vi "pumonarytesting_auto.vi"() -> ()   [LabVIEW 2014]
uses:
  <vilib>/vision/NI_Vision_Development_Module.lvlib
  <instrlib>/KD Scientific 2XX Series/KD Scientific 2XX Series.lvlib
panel:
  in  "Number of Cycles":i32
  out "Status":T1
  in  "stop 2":bool
  out "Delivered Volume":dbl
  out "Units":string
  in  "number of steps":i32
  in  "Baud Rate (9600)":u32(ring)=9600 items=["300"=300, "1200"=1200, "2400"=2400, "4800"=4800, "9600"=9600]
  in  "Withdrawal Settings":T2={"Flow Rate (5)"=5.0, "Volume (10)"=10.0, "Volume Units (ml)"=enum."milliliters (ml)", "Rate Units (ml/min.)"=enum."milliliters per minute (ml/min.)"} {"Volume (10)" format="%#.3g"}
  in  "Diameter (8.75 mm)":dbl=8.75
  in  "Infusion Settings":T2={"Flow Rate (5)"=5.0, "Volume (10)"=10.0, "Volume Units (ml)"=enum."milliliters (ml)", "Rate Units (ml/min.)"=enum."milliliters per minute (ml/min.)"}
  in  "Address (0)":i32 format="%0.0f"
  in  "error in (no error)":errorcluster
  in  "VISA resource name":refnum<visa-resource-name>="COM1"
  in  "stop 4":bool
  in  "stop":bool
  out "Image":T3(plugin-control)
  out "Particle Measurements (Pixels) (Particle Analysis 1)":dbl[][](array[numeric]) format="%.2f"
  out "subarray":dbl[](array[numeric])
  out "The diameter":dbl[](array[numeric])
  in  "stop (F)":bool
  out "Data from Transducer":dynamicdata(graph) caption="Voltage from Transducer V"
  out "Voltage from pressure transducer":dbl[](array[numeric])
  out "Pressure mm Hg":dbl[](graph)
  in  "Calibration factor":dbl[](array[numeric])
  in  "Zero Error":dbl[](array[numeric])
  out "pressure mm Hg":dbl[](array[numeric])
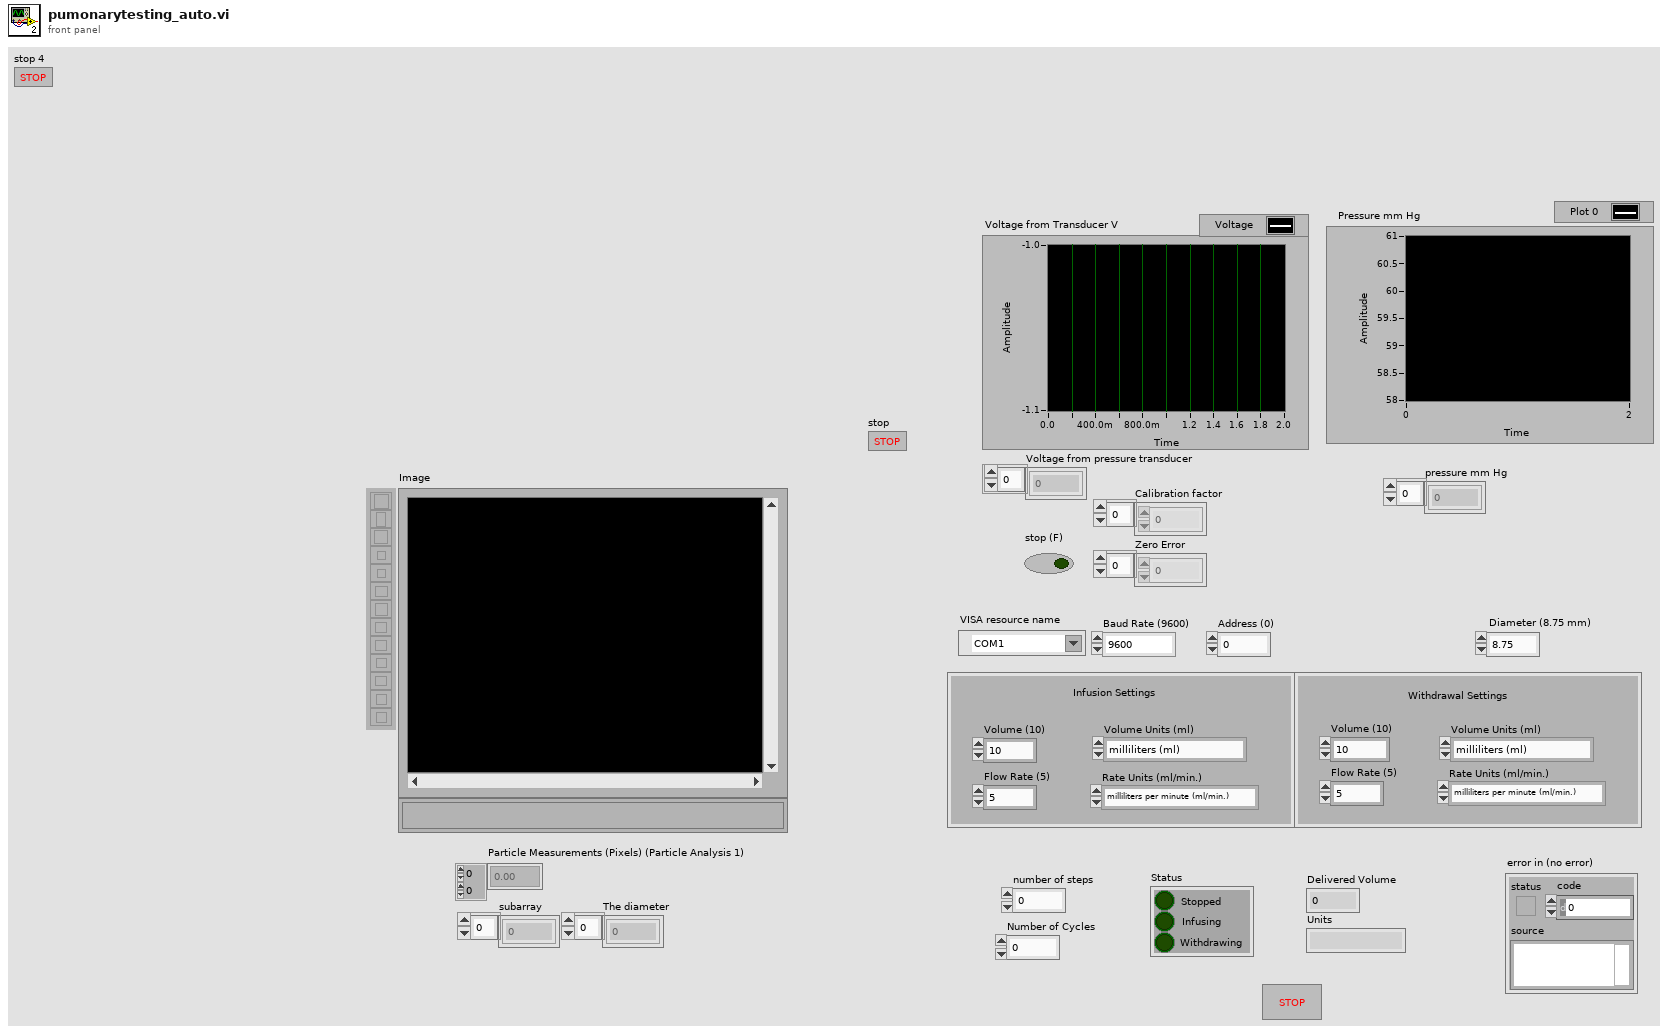
[diagram p1: front panel]
types:
  T1 = cluster{"Stopped":bool, "Infusing":bool, "Withdrawing":bool}
  T2 = cluster{"Flow Rate (5)":dbl, "Volume (10)":dbl, "Volume Units (ml)":enum16{"milliliters (ml)", "microliters (ul)"}, "Rate Units (ml/min.)":enum16{"milliliters per minute (ml/min.)", "milliliters per hour (ml/hr.)", "microliters per minute (ul/min.)", "microliters per hour (ul/hr.)"}}
  T3 = typedef "IMAQ Image.ctl" = refnum<image>
  T4 = typedef "Board Id" = u8
  T5 = typedef "ROI Descriptor" = cluster{"Global Rectangle":i32[], "Contours":cluster{"ID":enum32{"External", "Internal"}, "Type":u32, "Coordinates":i32[]}[]}
  T6 = enum16{"milliliters per minute (ml/min.)", "milliliters per hour (ml/hr.)", "microliters per minute (ul/min.)", "microliters per hour (ul/hr.)"}
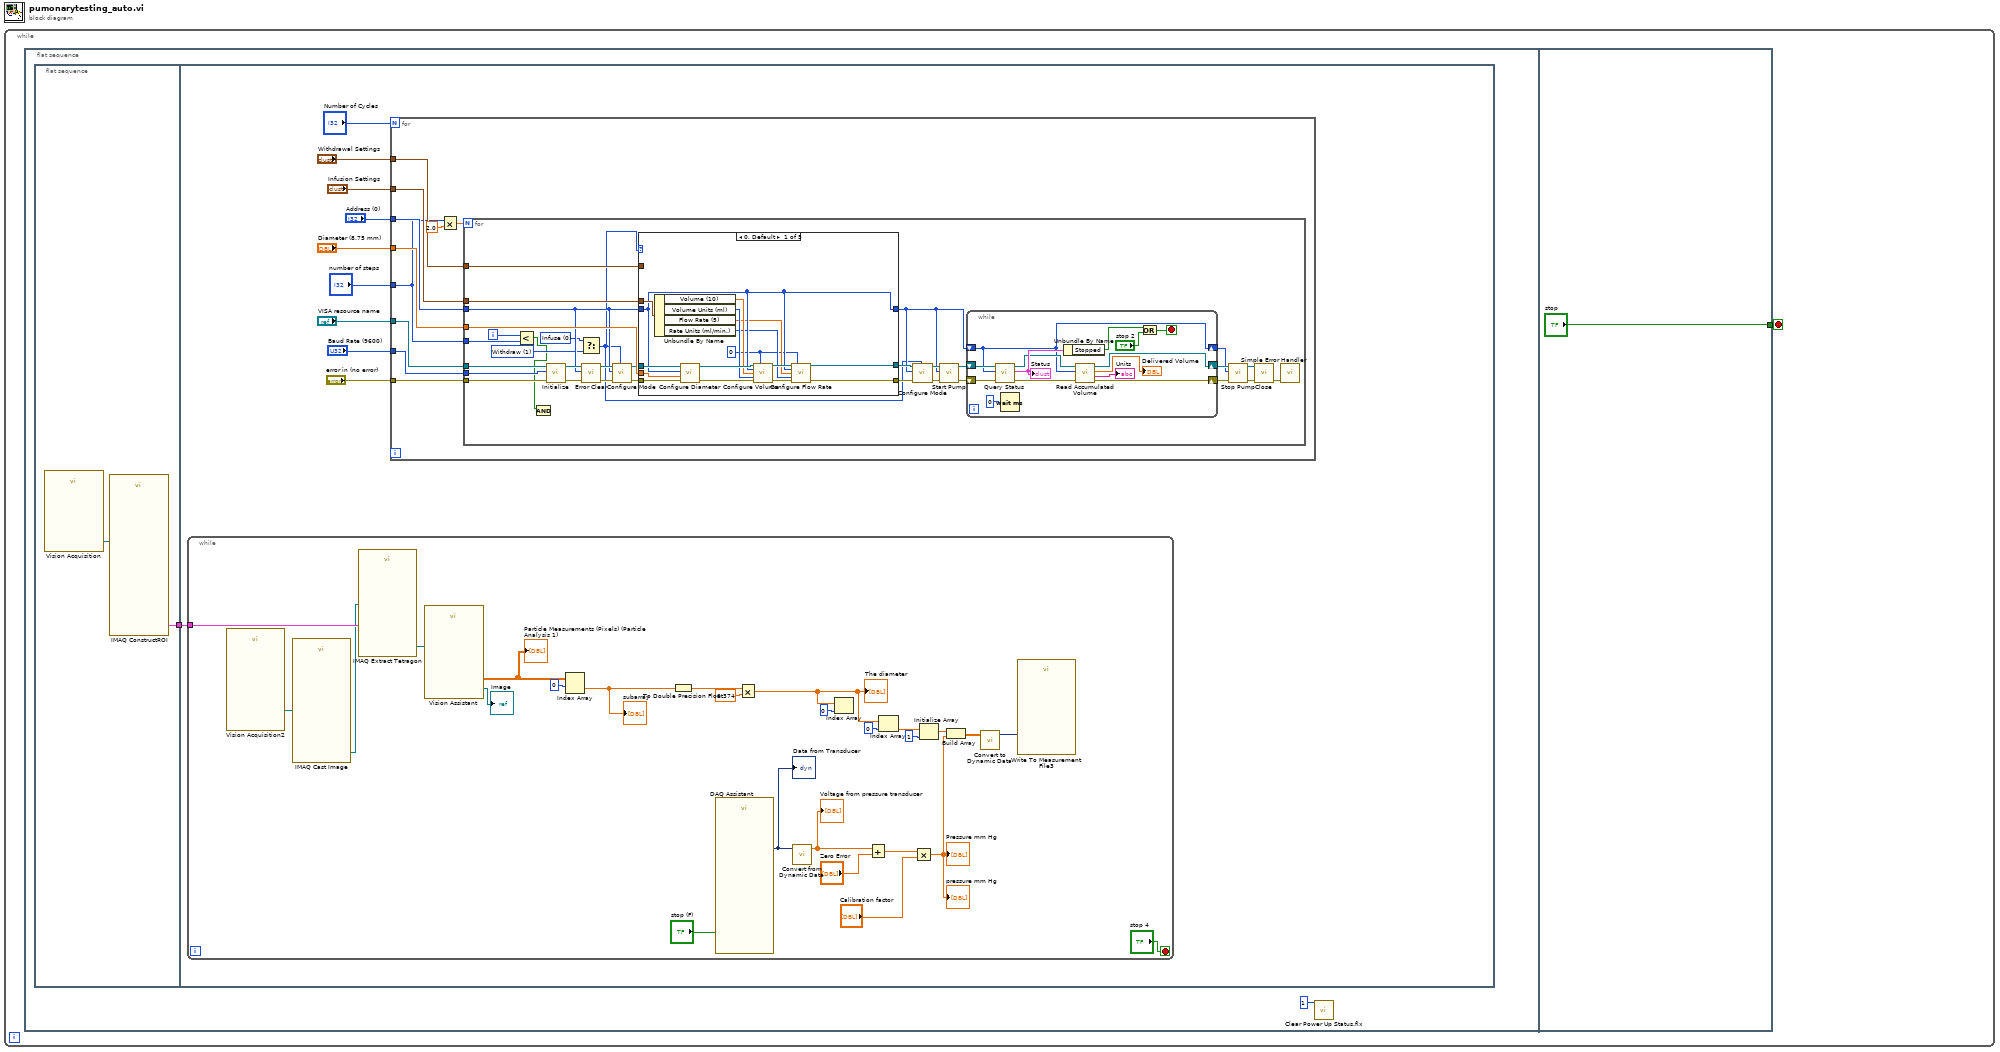
[diagram p0: block diagram]
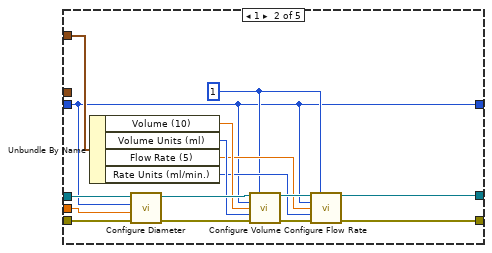
[diagram p2: hidden frame]
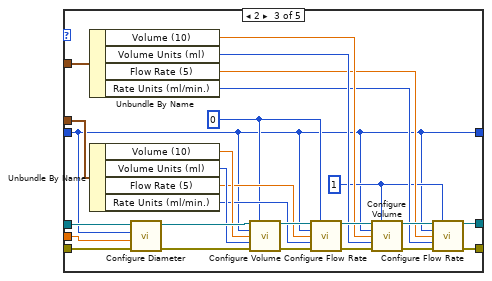
[diagram p3: hidden frame]
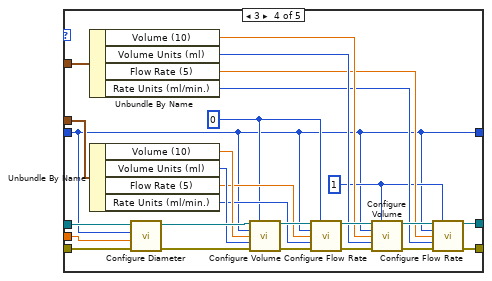
[diagram p4: hidden frame]
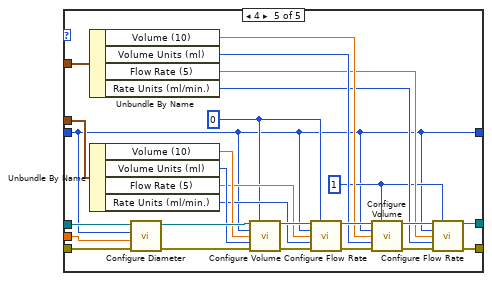
[diagram p5: hidden frame]
diagram:
  n1 = while {
    stop <- w1 stop-if-true
    n2 = flat-sequence {
      tunnel: ["stop"] -> w1
      frame #0 {
        n3 = flat-sequence {
          tunnel: [w4] -> w3
          tunnel: w3 -> [w15]
          frame #0 {
            n4 = call "Vision Acquisition"() -> ("Image Out"=w5:T3)  [unwired: 26 in, 1 out]
            n5 = call "IMAQ ConstructROI"("Image"=w5) -> ("ROI Descriptor Out"=w4:T5)  [unwired: 7 in, 3 out]
          }
          frame #1 {
            n6 = while {
              tunnel: w15 -> [w207]
              stop <- "stop 4" stop-if-true
              n7 = call "Vision Acquisition2"() -> ("Image Out"=w191:T3)  [unwired: 25 in, 2 out]
              n8 = call "IMAQ Cast Image"("Image Src"=w191) -> ("Image Dst Out"=w198:T3)  [unwired: 9 in, 1 out]
              n9 = call-poly "IMAQ Extract Tetragon"("ROI Descriptor"=w207, "Image Src"=w198) -> ("Image Dst Out"=w199:T3)  [unwired: 8 in, 1 out]
              n10 = call "Vision Assistant"("Image In"=w199) -> ("Image Out"=→"Image":T3, "Particle Measurements (Pixels) (Particle Analysis 1)"=w197:dbl[][])  [unwired: 23 in, 2 out]
              "Particle Measurements (Pixels) (Particle Analysis 1)" <- w197
              n11 = Index Array(array=w197, index (row)=0) -> (element=w195:dbl[])  [unwired: 1 in]
              "subarray" <- w195
              n12 = To Double Precision Float(number=w195) -> (double precision float=w194:dbl[])
              n13 = call "DAQ Assistant"("stop (F)"="stop (F)") -> ("data"=w206:dynamicdata)  [unwired: 15 in, 3 out]
              "Data from Transducer" <- w206
              n14 = Multiply(x=w194, y=0.374) -> (x*y=w187:dbl[])
              "The diameter" <- w187
              n15 = call "Convert from Dynamic Data"("Dynamic Data Type"=w206) -> ("Array"=w203:dbl[])  [unwired: 3 in]
              "Voltage from pressure transducer" <- w203
              n16 = Index Array(array=w187, index=0) -> ()  [unwired: 1 out]
              n17 = Add(x=w203, y="Zero Error") -> (x+y=w205:dbl[])
              n18 = Index Array(array=w187, index=0) -> (element=w186:dbl)
              n19 = Multiply(x=w205, y="Calibration factor") -> (x*y=w189:dbl[])
              "Pressure mm Hg" <- w189
              "pressure mm Hg" <- w189
              n20 = Initialize Array(w186, 1 ("dimension size")) -> (w184:dbl[])
              n21 = Build Array(w184, w189) -> (w183:dbl[][])
              n22 = call "Convert to Dynamic Data"("2D Array"=w183) -> ("Dynamic Data Type"=w182:dynamicdata)  [unwired: 3 in]
              n23 = call "Write To Measurement File3"("Signals"=w182) -> ()  [unwired: 16 in, 3 out]
            }
            n24 = for {
              N: "Number of Cycles" -> [_]
              tunnel: "VISA resource name" -> [w25]
              tunnel: "error in (no error)" -> [w24]
              tunnel: "Infusion Settings" -> [w23]
              tunnel: "Withdrawal Settings" -> [w22]
              tunnel: "Diameter (8.75 mm)" -> [w21]
              tunnel: "Baud Rate (9600)" -> [w20]
              tunnel: "Address (0)" -> [w19]
              tunnel: "number of steps" -> [w16]
              n25 = Multiply(x=w16, y=2.0) -> (x*y=w17:dbl)
              n26 = for {
                N: w17 -> [_]
                tunnel: w25 -> [w57]
                tunnel: w24 -> [w56]
                tunnel: w23 -> [w51]
                tunnel: w22 -> [w50]
                tunnel: w21 -> [w49]
                tunnel: w20 -> [w44]
                tunnel: w19 -> [w32]
                tunnel: w16 -> [w30]
                i -> [w31]
                w28 = u16 1 items=["Withdraw"=1]
                w29 = u16 0 items=["Infuse"] ("Mode (infuse)")
                n27 = Less?(x=w31, y=w30) -> (x < y?=w26:bool)
                n28 = And(x=w26) -> ()  [unwired: 1 in, 1 out]
                n29 = call <instrlib>:"Initialize.vi"("error in (no error)"=w56, "Baud Rate (9600)"=w44, "VISA resource name"=w57) -> ("error out"=w34:errorcluster, "VISA resource name out"=w33:refnum<visa-resource-name>)  [unwired: 7 in]
                n30 = Select(t=w29, f=w28) -> (s? t:f=w27:u16)  [unwired: 1 in]
                n31 = call <instrlib>:"Error Clear.vi"("error in (no error)"=w34, "Address (0)"=w32, "VISA resource name"=w33) -> ("error out"=w35:errorcluster, "VISA resource name out"=w36:refnum<visa-resource-name>)  [unwired: 6 in, 1 out]
                n32 = call <instrlib>:"Configure Mode.vi"("Mode (infuse)"=w27, "error in (no error)"=w35, "Address (0)"=w32, "VISA resource name"=w36) -> ("error out"=w38:errorcluster, "VISA resource name out"=w37:refnum<visa-resource-name>)  [unwired: 6 in]
                n33 = case shown="0, Default" w27 {
                  tunnel: w51 -> [w67 _ w115 w141 w167]
                  tunnel: w50 -> [_ w89 w114 w140 w166]
                  tunnel: w37 -> [w73 w88 w113 w139 w165]
                  tunnel: w38 -> [w72 w84 w112 w138 w164]
                  tunnel: w49 -> [w66 w80 w95 w121 w147]
                  tunnel: [w65 w74 w90 w116 w142] -> w39
                  tunnel: w32 -> [w65 w74 w90 w116 w142]
                  tunnel: [w60 w85 w92 w118 w144] -> w43
                  tunnel: [w59 w81 w91 w117 w143] -> w42
                  frame 0, Default {
                    w58 = 0
                    n34 = Unbundle By Name(w67) -> ("Volume (10)"=w64:dbl, "Volume Units (ml)"=w63:enum16{"milliliters (ml)", "microliters (ul)"}, "Flow Rate (5)"=w62:dbl, "Rate Units (ml/min.)"=w61:T6)
                    n35 = call <instrlib>:"Configure Diameter.vi"("error in (no error)"=w72, "Diameter (8.75 mm)"=w66, "Address (0)"=w65, "VISA resource name"=w73) -> ("error out"=w70:errorcluster, "VISA resource name out"=w71:refnum<visa-resource-name>)  [unwired: 6 in]
                    n36 = call <instrlib>:"Configure Volume.vi"("VISA resource name"=w71, "Mode (infuse)"=w58, "Address (0)"=w65, "Volume (100)"=w64, "Units (0: milliliters)"=w63, "error in (no error)"=w70) -> ("VISA resource name out"=w69:refnum<visa-resource-name>, "error out"=w68:errorcluster)  [unwired: 8 in]
                    n37 = call <instrlib>:"Configure Flow Rate.vi"("VISA resource name"=w69, "Mode (infuse)"=w58, "Address (0)"=w65, "Flow Rate (5)"=w62, "Units (0: milliliters per minute)"=w61, "error in (no error)"=w68) -> ("VISA resource name out"=w60:refnum<visa-resource-name>, "error out"=w59:errorcluster)  [unwired: 8 in]
                  }
                  frame 1 {
                    w75 = 1
                    n38 = Unbundle By Name(w89) -> ("Volume (10)"=w79:dbl, "Volume Units (ml)"=w78:enum16{"milliliters (ml)", "microliters (ul)"}, "Flow Rate (5)"=w77:dbl, "Rate Units (ml/min.)"=w76:T6)
                    n39 = call <instrlib>:"Configure Diameter.vi"("error in (no error)"=w84, "Diameter (8.75 mm)"=w80, "Address (0)"=w74, "VISA resource name"=w88) -> ("error out"=w83:errorcluster, "VISA resource name out"=w87:refnum<visa-resource-name>)  [unwired: 6 in]
                    n40 = call <instrlib>:"Configure Volume.vi"("VISA resource name"=w87, "Mode (infuse)"=w75, "Address (0)"=w74, "Volume (100)"=w79, "Units (0: milliliters)"=w78, "error in (no error)"=w83) -> ("VISA resource name out"=w86:refnum<visa-resource-name>, "error out"=w82:errorcluster)  [unwired: 8 in]
                    n41 = call <instrlib>:"Configure Flow Rate.vi"("VISA resource name"=w86, "Mode (infuse)"=w75, "Address (0)"=w74, "Flow Rate (5)"=w77, "Units (0: milliliters per minute)"=w76, "error in (no error)"=w82) -> ("VISA resource name out"=w85:refnum<visa-resource-name>, "error out"=w81:errorcluster)  [unwired: 8 in]
                  }
                  frame 2 {
                    w93 = 1
                    w94 = 0
                    n42 = Unbundle By Name(w114) -> ("Volume (10)"=w99:dbl, "Volume Units (ml)"=w98:enum16{"milliliters (ml)", "microliters (ul)"}, "Flow Rate (5)"=w97:dbl, "Rate Units (ml/min.)"=w96:T6)
                    n43 = Unbundle By Name(w115) -> ("Volume (10)"=w103:dbl, "Volume Units (ml)"=w102:enum16{"milliliters (ml)", "microliters (ul)"}, "Flow Rate (5)"=w101:dbl, "Rate Units (ml/min.)"=w100:T6)
                    n44 = call <instrlib>:"Configure Diameter.vi"("error in (no error)"=w112, "Diameter (8.75 mm)"=w95, "Address (0)"=w90, "VISA resource name"=w113) -> ("error out"=w107:errorcluster, "VISA resource name out"=w111:refnum<visa-resource-name>)  [unwired: 6 in]
                    n45 = call <instrlib>:"Configure Volume.vi"("VISA resource name"=w111, "Mode (infuse)"=w94, "Address (0)"=w90, "Volume (100)"=w103, "Units (0: milliliters)"=w102, "error in (no error)"=w107) -> ("VISA resource name out"=w110:refnum<visa-resource-name>, "error out"=w106:errorcluster)  [unwired: 8 in]
                    n46 = call <instrlib>:"Configure Flow Rate.vi"("VISA resource name"=w110, "Mode (infuse)"=w94, "Address (0)"=w90, "Flow Rate (5)"=w101, "Units (0: milliliters per minute)"=w100, "error in (no error)"=w106) -> ("VISA resource name out"=w109:refnum<visa-resource-name>, "error out"=w105:errorcluster)  [unwired: 8 in]
                    n47 = call <instrlib>:"Configure Volume.vi"("VISA resource name"=w109, "Mode (infuse)"=w93, "Address (0)"=w90, "Volume (100)"=w99, "Units (0: milliliters)"=w98, "error in (no error)"=w105) -> ("VISA resource name out"=w108:refnum<visa-resource-name>, "error out"=w104:errorcluster)  [unwired: 8 in]
                    n48 = call <instrlib>:"Configure Flow Rate.vi"("VISA resource name"=w108, "Mode (infuse)"=w93, "Address (0)"=w90, "Flow Rate (5)"=w97, "Units (0: milliliters per minute)"=w96, "error in (no error)"=w104) -> ("VISA resource name out"=w92:refnum<visa-resource-name>, "error out"=w91:errorcluster)  [unwired: 8 in]
                  }
                  frame 3 {
                    w119 = 1
                    w120 = 0
                    n49 = Unbundle By Name(w140) -> ("Volume (10)"=w125:dbl, "Volume Units (ml)"=w124:enum16{"milliliters (ml)", "microliters (ul)"}, "Flow Rate (5)"=w123:dbl, "Rate Units (ml/min.)"=w122:T6)
                    n50 = Unbundle By Name(w141) -> ("Volume (10)"=w129:dbl, "Volume Units (ml)"=w128:enum16{"milliliters (ml)", "microliters (ul)"}, "Flow Rate (5)"=w127:dbl, "Rate Units (ml/min.)"=w126:T6)
                    n51 = call <instrlib>:"Configure Diameter.vi"("error in (no error)"=w138, "Diameter (8.75 mm)"=w121, "Address (0)"=w116, "VISA resource name"=w139) -> ("error out"=w133:errorcluster, "VISA resource name out"=w137:refnum<visa-resource-name>)  [unwired: 6 in]
                    n52 = call <instrlib>:"Configure Volume.vi"("VISA resource name"=w137, "Mode (infuse)"=w120, "Address (0)"=w116, "Volume (100)"=w129, "Units (0: milliliters)"=w128, "error in (no error)"=w133) -> ("VISA resource name out"=w136:refnum<visa-resource-name>, "error out"=w132:errorcluster)  [unwired: 8 in]
                    n53 = call <instrlib>:"Configure Flow Rate.vi"("VISA resource name"=w136, "Mode (infuse)"=w120, "Address (0)"=w116, "Flow Rate (5)"=w127, "Units (0: milliliters per minute)"=w126, "error in (no error)"=w132) -> ("VISA resource name out"=w135:refnum<visa-resource-name>, "error out"=w131:errorcluster)  [unwired: 8 in]
                    n54 = call <instrlib>:"Configure Volume.vi"("VISA resource name"=w135, "Mode (infuse)"=w119, "Address (0)"=w116, "Volume (100)"=w125, "Units (0: milliliters)"=w124, "error in (no error)"=w131) -> ("VISA resource name out"=w134:refnum<visa-resource-name>, "error out"=w130:errorcluster)  [unwired: 8 in]
                    n55 = call <instrlib>:"Configure Flow Rate.vi"("VISA resource name"=w134, "Mode (infuse)"=w119, "Address (0)"=w116, "Flow Rate (5)"=w123, "Units (0: milliliters per minute)"=w122, "error in (no error)"=w130) -> ("VISA resource name out"=w118:refnum<visa-resource-name>, "error out"=w117:errorcluster)  [unwired: 8 in]
                  }
                  frame 4 {
                    w145 = 1
                    w146 = 0
                    n56 = Unbundle By Name(w166) -> ("Volume (10)"=w151:dbl, "Volume Units (ml)"=w150:enum16{"milliliters (ml)", "microliters (ul)"}, "Flow Rate (5)"=w149:dbl, "Rate Units (ml/min.)"=w148:T6)
                    n57 = Unbundle By Name(w167) -> ("Volume (10)"=w155:dbl, "Volume Units (ml)"=w154:enum16{"milliliters (ml)", "microliters (ul)"}, "Flow Rate (5)"=w153:dbl, "Rate Units (ml/min.)"=w152:T6)
                    n58 = call <instrlib>:"Configure Diameter.vi"("error in (no error)"=w164, "Diameter (8.75 mm)"=w147, "Address (0)"=w142, "VISA resource name"=w165) -> ("error out"=w159:errorcluster, "VISA resource name out"=w163:refnum<visa-resource-name>)  [unwired: 6 in]
                    n59 = call <instrlib>:"Configure Volume.vi"("VISA resource name"=w163, "Mode (infuse)"=w146, "Address (0)"=w142, "Volume (100)"=w155, "Units (0: milliliters)"=w154, "error in (no error)"=w159) -> ("VISA resource name out"=w162:refnum<visa-resource-name>, "error out"=w158:errorcluster)  [unwired: 8 in]
                    n60 = call <instrlib>:"Configure Flow Rate.vi"("VISA resource name"=w162, "Mode (infuse)"=w146, "Address (0)"=w142, "Flow Rate (5)"=w153, "Units (0: milliliters per minute)"=w152, "error in (no error)"=w158) -> ("VISA resource name out"=w161:refnum<visa-resource-name>, "error out"=w157:errorcluster)  [unwired: 8 in]
                    n61 = call <instrlib>:"Configure Volume.vi"("VISA resource name"=w161, "Mode (infuse)"=w145, "Address (0)"=w142, "Volume (100)"=w151, "Units (0: milliliters)"=w150, "error in (no error)"=w157) -> ("VISA resource name out"=w160:refnum<visa-resource-name>, "error out"=w156:errorcluster)  [unwired: 8 in]
                    n62 = call <instrlib>:"Configure Flow Rate.vi"("VISA resource name"=w160, "Mode (infuse)"=w145, "Address (0)"=w142, "Flow Rate (5)"=w149, "Units (0: milliliters per minute)"=w148, "error in (no error)"=w156) -> ("VISA resource name out"=w144:refnum<visa-resource-name>, "error out"=w143:errorcluster)  [unwired: 8 in]
                  }
                }
                n63 = call <instrlib>:"Configure Mode.vi"("Mode (infuse)"=w27, "error in (no error)"=w42, "Address (0)"=w39, "VISA resource name"=w43) -> ("error out"=w40:errorcluster, "VISA resource name out"=w41:refnum<visa-resource-name>)  [unwired: 6 in]
                n64 = call <instrlib>:"Start Pump.vi"("error in (no error)"=w40, "Address (0)"=w39, "VISA resource name"=w41) -> ("error out"=w54:errorcluster, "VISA resource name out"=w55:refnum<visa-resource-name>)  [unwired: 7 in]
                n65 = while {
                  shift-right: [w170] -> w48
                  shift-left: w39 -> [w170]
                  shift-right: [w172] -> w53
                  shift-left: w55 -> [w178]
                  shift-right: [w171] -> w52
                  shift-left: w54 -> [w179]
                  stop <- w176 stop-if-true
                  n66 = call <instrlib>:"Query Status.vi"("error in (no error)"=w179, "Address (0)"=w170, "VISA resource name"=w178) -> ("error out"=w181:errorcluster, "Status"=w177:T1, "VISA resource name out"=w173:refnum<visa-resource-name>)  [unwired: 6 in]
                  "Status" <- w177
                  n67 = Wait (ms)(milliseconds to wait=u32 0) -> ()  [unwired: 1 out]
                  n68 = Unbundle By Name(w177) -> ("Stopped"=w175:bool)
                  n69 = call <instrlib>:"Read Accumulated Volume.vi"("error in (no error)"=w181, "Address (0)"=w170, "VISA resource name"=w173) -> ("error out"=w171:errorcluster, "Units"=→"Units":string, "Delivered Volume"=→"Delivered Volume":dbl, "VISA resource name out"=w172:refnum<visa-resource-name>)  [unwired: 5 in]
                  n70 = Or(x=w175, y="stop 2") -> (x .or. y?=w176:bool)
                }
                n71 = call <instrlib>:"Stop Pump.vi"("error in (no error)"=w52, "Address (0)"=w48, "VISA resource name"=w53) -> ("error out"=w46:errorcluster, "VISA resource name out"=w45:refnum<visa-resource-name>)  [unwired: 7 in]
                n72 = call <instrlib>:"Close.vi"("error in (no error)"=w46, "VISA resource name"=w45) -> ("error out"=w47:errorcluster)  [unwired: 9 in]
                n73 = call <vilib>:"Simple Error Handler.vi"("error in (no error)"=w47) -> ()  [unwired: 4 in, 5 out]
              }
            }
          }
        }
        n74 = call <vilib>:"Clear Power Up Status.flx"("Board ID"=T4 1) -> ()  [unwired: 6 in, 2 out]
      }
      frame #1 {
      }
    }
  }
